vi "UHR-Fleezers Control (host) - Lorentz v4.vi"() -> ()   [LabVIEW 2014] (continued)
                                n2618 = Multiply(x=w4043, y=1000.0) -> (x*y=w4041:dbl)
                                n2619 = Wait (ms)(milliseconds to wait=w4041) -> ()  [unwired: 1 out]
                                }
                                frame #1 {
                                n2620 = local read "Yank to which?"() -> (w4045:bool)
                                n2621 = local read "Random Choice"() -> (w4055:bool)
                                n2622 = local read "Yank to Trap Delta (MHz)"() -> (w4048:dbl[])
                                n2623 = local read "Yank to SP"() -> (w4049:dbl[])
                                n2624 = Random Number (0-1)() -> (number: 0 to 1=w4054:dbl)
                                n2625 = Multiply(x=w4051, y=w4054) -> (x*y=w4053:dbl)
                                n2626 = Round Toward -Infinity(1:w4053) -> (0:w4052:dbl)
                                n2627 = Select(t=w4052, s=w4055, f=w4050) -> (s? t:f=w4046:dbl)
                                n2628 = Select(t=w4048, s=w4045, f=w4049) -> (s? t:f=w4047:dbl[])
                                n2629 = Index Array(array=w4047, index=w4046) -> (element=w4044:dbl)
                                n2630 = case shown="True" w4045 {
                                tunnel: w4044 -> [w4056 w4083]
                                frame False {
                                n2631 = flat-sequence {
                                tunnel: w4056 -> [w4057]
                                frame #0 {
                                n2632 = property on="Trap Pos FB SP" class="DigNum (strict)"("Val(Sgnl)"=w4057) -> ()  [unwired: 2 in, 2 out]
                                }
                                frame #1 {
                                n2633 = Wait (ms)(milliseconds to wait=u32 700) -> ()  [unwired: 1 out]
                                }
                                frame #2 {
                                n2634 = local read "Action (%)"() -> (w4062:dbl)
                                n2635 = Absolute Value(x=w4062) -> (abs(x)=w4061:dbl)
                                n2636 = Greater?(x=w4061, y=70.0) -> (0:w4059:bool)
                                n2637 = property on="Remove Action Offset" class="Bool (strict)"("Val(Sgnl)"=w4059) -> ()  [unwired: 2 in, 2 out]
                                }
                                frame #3 {
                                n2638 = for {
                                N: 4 -> [_]
                                n2639 = flat-sequence {
                                frame #0 {
                                n2640 = Wait (ms)(milliseconds to wait=u32 500) -> ()  [unwired: 1 out]
                                }
                                frame #1 {
                                n2641 = local read "Action (%)"() -> (w4068:dbl)
                                n2642 = Absolute Value(x=w4068) -> (abs(x)=w4067:dbl)
                                n2643 = Greater?(x=w4067, y=70.0) -> (0:w4065:bool)
                                n2644 = property on="Remove Action Offset" class="Bool (strict)"("Val(Sgnl)"=w4065) -> ()  [unwired: 2 in, 2 out]
                                }
                                }
                                }
                                }
                                frame #4 {
                                n2645 = Wait (ms)(milliseconds to wait=u32 500) -> ()  [unwired: 1 out]
                                }
                                frame #5 {
                                n2646 = local read "Mean"() -> (w4076:dbl)
                                n2647 = Greater?(x=w4076, y=11.0) -> (0:w4070:bool)
                                n2648 = Not(x=w4070) -> (.not. x?=w4071:bool)
                                n2649 = And(x=w4071, y="Shift confocal") -> (x .and. y?=w4073:bool)
                                n2650 = And(x=w4070, y="Shift confocal") -> (x .and. y?=w4074:bool)
                                n2651 = case shown="True" w4074 {
                                frame False {
                                }
                                frame True {
                                n2652 = local read "Confocal Y 2 (V)"() -> (w4080:dbl)
                                n2653 = local read "Confocal X 2 (V)"() -> (w4079:dbl)
                                n2654 = property on="AO1" class="Slide (strict)"("Val(Sgnl)"=w4080) -> ()  [unwired: 2 in, 2 out]
                                n2655 = property on="AO2" class="Slide (strict)"("Val(Sgnl)"=w4079) -> ()  [unwired: 2 in, 2 out]
                                }
                                }
                                n2656 = case shown="True" w4073 {
                                frame False {
                                }
                                frame True {
                                n2657 = local read "Confocal Y 1 (V)"() -> (w4078:dbl)
                                n2658 = local read "Confocal X 1 (V)"() -> (w4077:dbl)
                                n2659 = property on="AO1" class="Slide (strict)"("Val(Sgnl)"=w4078) -> ()  [unwired: 2 in, 2 out]
                                n2660 = property on="AO2" class="Slide (strict)"("Val(Sgnl)"=w4077) -> ()  [unwired: 2 in, 2 out]
                                }
                                }
                                }
                                frame #6 {
                                n2661 = Wait (ms)(milliseconds to wait=u32 1500) -> ()  [unwired: 1 out]
                                }
                                frame #7 {
                                n2662 = property on="Rem fb disp offset" class="Bool (strict)"("Val(Sgnl)"=TRUE ("Value (Signaling)")) -> ()  [unwired: 2 in, 2 out]
                                }
                                }
                                }
                                frame True {
                                n2663 = flat-sequence {
                                tunnel: w4083 -> [w4084]
                                frame #0 {
                                n2664 = property on="Trap Delta (MHz)" class="DigNum (strict)"("Val(Sgnl)"=w4084) -> ()  [unwired: 2 in, 2 out]
                                }
                                frame #1 {
                                n2665 = Wait (ms)(milliseconds to wait=u32 500) -> ()  [unwired: 1 out]
                                }
                                frame #2 {
                                n2666 = local read "Shift confocal"() -> (w4090:bool)
                                n2667 = local read "Mean"() -> (w4092:dbl)
                                n2668 = Greater?(x=w4092, y=11.0) -> (0:w4089:bool)
                                n2669 = Not(x=w4089) -> (.not. x?=w4088:bool)
                                n2670 = And(x=w4088, y=w4090) -> (x .and. y?=w4086:bool)
                                n2671 = And(x=w4089, y=w4090) -> (x .and. y?=w4087:bool)
                                n2672 = case shown="True" w4087 {
                                frame False {
                                }
                                frame True {
                                n2673 = local read "Confocal Y 2 (V)"() -> (w4096:dbl)
                                n2674 = local read "Confocal X 2 (V)"() -> (w4095:dbl)
                                n2675 = property on="AO2" class="Slide (strict)"("Val(Sgnl)"=w4095) -> ()  [unwired: 2 in, 2 out]
                                n2676 = property on="AO1" class="Slide (strict)"("Val(Sgnl)"=w4096) -> ()  [unwired: 2 in, 2 out]
                                }
                                }
                                n2677 = case shown="True" w4086 {
                                frame False {
                                }
                                frame True {
                                n2678 = local read "Confocal X 1 (V)"() -> (w4093:dbl)
                                n2679 = local read "Confocal Y 1 (V)"() -> (w4094:dbl)
                                n2680 = property on="AO2" class="Slide (strict)"("Val(Sgnl)"=w4093) -> ()  [unwired: 2 in, 2 out]
                                n2681 = property on="AO1" class="Slide (strict)"("Val(Sgnl)"=w4094) -> ()  [unwired: 2 in, 2 out]
                                }
                                }
                                }
                                }
                                }
                                }
                                }
                                }
                                }
                                frame "Image" {
                                n2682 = property on="Confocal Image" class="Bool (strict)"("Val(Sgnl)"=TRUE ("Value (Signaling)")) -> ()  [unwired: 2 in, 2 out]
                                }
                              }
                              n2683 = local write "Fl. High"(FALSE ("Fl. High")) -> ()
                              n2684 = local read "Time (s)"() -> (w4030:dbl)
                            }
                            frame #1 {
                              n2685 = case shown="True" "Auto F Reset" {
                                tunnel: w4102 -> [_ w4107]
                                tunnel: w4101 -> [_ w4106]
                                tunnel: w4100 -> [_ w4105]
                                tunnel: w4099 -> [_ w4104]
                                frame False {
                                }
                                frame True {
                                n2686 = node-c288() -> (w4109:T35)  [unwired: 4 in]
                                n2687 = timed-loop {
                                timing: w4109 -> [_]
                                timing-out: [_] -> w4108
                                tunnel: w4107 -> [w4114]
                                tunnel: w4106 -> [w4113]
                                tunnel: w4105 -> [w4112]
                                tunnel: w4104 -> [w4111]
                                stop <- w4110 stop-if-true
                                n2688 = node-c288() -> ()  [unwired: 1 in, 1 out]
                                n2689 = local read "Fl. Delta Thresh. (kHz)"() -> (w4123:dbl)
                                n2690 = local read "APD to Watch"() -> (w4124:bool)
                                n2691 = local read "Delta Fl. 1"() -> (w4125:dbl)
                                n2692 = local read "Delta Fl. 2"() -> (w4126:dbl)
                                n2693 = local read "Fl. Triggered..."() -> (w4117:bool)
                                n2694 = local read "Stop All"() -> (w4118:bool)
                                n2695 = local read "Reset Force"() -> (w4116:bool)
                                n2696 = Multiply(x=w4123, y=1000.0) -> (x*y=w4121:dbl)
                                n2697 = Select(t=w4125, s=w4124, f=w4126) -> (s? t:f=w4120:dbl)
                                n2698 = Not(x=w4117) -> (.not. x?=w4115:bool)
                                n2699 = Greater?(x=w4120, y=w4121) -> (0:w4119:bool)
                                n2700 = Compound Arithmetic op=OR(w4119, w4118, w4115, w4116) -> (w4110:bool)
                                n2701 = case shown="True" w4110 {
                                tunnel: w4114 -> [_ w4130]
                                tunnel: w4113 -> [_ w4134]
                                tunnel: w4112 -> [_ w4133]
                                tunnel: w4111 -> [_ w4132]
                                frame False {
                                }
                                frame True {
                                n2702 = case shown="\"Yank\"" w4134 {
                                tunnel: w4133 -> [_ w4144]
                                tunnel: w4132 -> [_ w4142]
                                frame "Image", Default {
                                }
                                frame "Yank" {
                                n2703 = flat-sequence {
                                tunnel: [w4147] -> w4145
                                tunnel: w4144 -> [w4147]
                                tunnel: [w4146] -> w4143
                                tunnel: w4142 -> [w4146]
                                tunnel: w4145 -> [w4153]
                                tunnel: w4143 -> [w4151]
                                frame #0 {
                                n2704 = local read "Yank Delay (s)"() -> (w4150:dbl)
                                n2705 = Multiply(x=w4150, y=1000.0) -> (x*y=w4148:dbl)
                                n2706 = Wait (ms)(milliseconds to wait=w4148) -> ()  [unwired: 1 out]
                                }
                                frame #1 {
                                n2707 = local read "Yank to which?"() -> (w4152:bool)
                                n2708 = case shown="False" w4152 {
                                tunnel: w4153 -> [_ w4181]
                                tunnel: w4151 -> [w4154 _]
                                frame False {
                                n2709 = flat-sequence {
                                tunnel: w4154 -> [w4155]
                                frame #0 {
                                n2710 = property on="Trap Pos FB SP" class="DigNum (strict)"("Val(Sgnl)"=w4155) -> ()  [unwired: 2 in, 2 out]
                                }
                                frame #1 {
                                n2711 = Wait (ms)(milliseconds to wait=u32 700) -> ()  [unwired: 1 out]
                                }
                                frame #2 {
                                n2712 = local read "Action (%)"() -> (w4160:dbl)
                                n2713 = Absolute Value(x=w4160) -> (abs(x)=w4159:dbl)
                                n2714 = Greater?(x=w4159, y=70.0) -> (0:w4157:bool)
                                n2715 = property on="Remove Action Offset" class="Bool (strict)"("Val(Sgnl)"=w4157) -> ()  [unwired: 2 in, 2 out]
                                }
                                frame #3 {
                                n2716 = for {
                                N: 4 -> [_]
                                n2717 = flat-sequence {
                                frame #0 {
                                n2718 = Wait (ms)(milliseconds to wait=u32 500) -> ()  [unwired: 1 out]
                                }
                                frame #1 {
                                n2719 = local read "Action (%)"() -> (w4166:dbl)
                                n2720 = Absolute Value(x=w4166) -> (abs(x)=w4165:dbl)
                                n2721 = Greater?(x=w4165, y=70.0) -> (0:w4163:bool)
                                n2722 = property on="Remove Action Offset" class="Bool (strict)"("Val(Sgnl)"=w4163) -> ()  [unwired: 2 in, 2 out]
                                }
                                }
                                }
                                }
                                frame #4 {
                                n2723 = Wait (ms)(milliseconds to wait=u32 500) -> ()  [unwired: 1 out]
                                }
                                frame #5 {
                                n2724 = local read "Shift confocal"() -> (w4171:bool)
                                n2725 = local read "Mean"() -> (w4174:dbl)
                                n2726 = Greater?(x=w4174, y=11.0) -> (0:w4170:bool)
                                n2727 = Not(x=w4170) -> (.not. x?=w4169:bool)
                                n2728 = And(x=w4170, y=w4171) -> (x .and. y?=w4172:bool)
                                n2729 = And(x=w4169, y=w4171) -> (x .and. y?=w4168:bool)
                                n2730 = case shown="True" w4172 {
                                frame False {
                                }
                                frame True {
                                n2731 = local read "Confocal X 2 (V)"() -> (w4177:dbl)
                                n2732 = local read "Confocal Y 2 (V)"() -> (w4178:dbl)
                                n2733 = property on="AO2" class="Slide (strict)"("Val(Sgnl)"=w4177) -> ()  [unwired: 2 in, 2 out]
                                n2734 = property on="AO1" class="Slide (strict)"("Val(Sgnl)"=w4178) -> ()  [unwired: 2 in, 2 out]
                                }
                                }
                                n2735 = case shown="True" w4168 {
                                frame False {
                                }
                                frame True {
                                n2736 = local read "Confocal Y 1 (V)"() -> (w4176:dbl)
                                n2737 = local read "Confocal X 1 (V)"() -> (w4175:dbl)
                                n2738 = property on="AO1" class="Slide (strict)"("Val(Sgnl)"=w4176) -> ()  [unwired: 2 in, 2 out]
                                n2739 = property on="AO2" class="Slide (strict)"("Val(Sgnl)"=w4175) -> ()  [unwired: 2 in, 2 out]
                                }
                                }
                                }
                                frame #6 {
                                n2740 = Wait (ms)(milliseconds to wait=u32 1500) -> ()  [unwired: 1 out]
                                }
                                frame #7 {
                                n2741 = property on="Rem fb disp offset" class="Bool (strict)"("Val(Sgnl)"=TRUE ("Value (Signaling)")) -> ()  [unwired: 2 in, 2 out]
                                }
                                }
                                }
                                frame True {
                                n2742 = flat-sequence {
                                tunnel: w4181 -> [w4182]
                                frame #0 {
                                n2743 = property on="Trap Delta (MHz)" class="DigNum (strict)"("Val(Sgnl)"=w4182) -> ()  [unwired: 2 in, 2 out]
                                }
                                frame #1 {
                                n2744 = Wait (ms)(milliseconds to wait=u32 500) -> ()  [unwired: 1 out]
                                }
                                frame #2 {
                                n2745 = local read "Shift confocal"() -> (w4188:bool)
                                n2746 = local read "Mean"() -> (w4189:dbl)
                                n2747 = Greater?(x=w4189, y=11.0) -> (0:w4187:bool)
                                n2748 = And(x=w4187, y=w4188) -> (x .and. y?=w4185:bool)
                                n2749 = Not(x=w4187) -> (.not. x?=w4186:bool)
                                n2750 = And(x=w4186, y=w4188) -> (x .and. y?=w4184:bool)
                                n2751 = case shown="True" w4185 {
                                frame False {
                                }
                                frame True {
                                n2752 = local read "Confocal Y 2 (V)"() -> (w4194:dbl)
                                n2753 = local read "Confocal X 2 (V)"() -> (w4193:dbl)
                                n2754 = property on="AO1" class="Slide (strict)"("Val(Sgnl)"=w4194) -> ()  [unwired: 2 in, 2 out]
                                n2755 = property on="AO2" class="Slide (strict)"("Val(Sgnl)"=w4193) -> ()  [unwired: 2 in, 2 out]
                                }
                                }
                                n2756 = case shown="True" w4184 {
                                frame False {
                                }
                                frame True {
                                n2757 = local read "Confocal Y 1 (V)"() -> (w4192:dbl)
                                n2758 = local read "Confocal X 1 (V)"() -> (w4191:dbl)
                                n2759 = property on="AO2" class="Slide (strict)"("Val(Sgnl)"=w4191) -> ()  [unwired: 2 in, 2 out]
                                n2760 = property on="AO1" class="Slide (strict)"("Val(Sgnl)"=w4192) -> ()  [unwired: 2 in, 2 out]
                                }
                                }
                                }
                                }
                                }
                                }
                                }
                                }
                                }
                                }
                                n2761 = local read "Time (s)"() -> (w4129:dbl)
                                n2762 = Subtract(x=w4130, y=w4129) -> (x-y=w4141:dbl)
                                n2763 = Number To Decimal String(number=w4141, width (-)=i16 0) -> (decimal integer string=w4139:string)
                                n2764 = Concatenate Strings(w4139, " s fluorescence event") -> (w4136:string)
                                n2765 = local read "Messages"() -> (w4137:string)
                                n2766 = local write "Duration (s)"(w4141) -> ()
                                n2767 = call "Update messages.vi"("Message to add"=w4136, "Old message string"=w4137) -> ("New message string"=w4135:string)
                                n2768 = local write "Messages"(w4135) -> ()
                                n2769 = call <vilib>:"Beep.vi"() -> ()  [unwired: 12 in]
                                n2770 = local write "Reset Force"(FALSE ("Force Reset")) -> ()
                                n2771 = local write "Fl. High"(TRUE ("Fl. High")) -> ()
                                n2772 = local write "Waiting"(TRUE ("Waiting")) -> ()
                                }
                                }
                                n2773 = node-c288() -> ()  [unwired: 1 in, 1 out]
                                }
                                n2774 = node-c288(w4108) -> ()  [unwired: 1 out]
                                }
                              }
                            }
                          }
                          n2775 = local read "Trap Delta (MHz)"() -> (w4020:dbl)
                          n2776 = local read "Trap Pos FB SP"() -> (w4018:fxp<+/-,16,1>)
                        }
                      }
                    }
                    frame True {
                      n2777 = flat-sequence {
                        tunnel: w4205 -> [w4215]
                        tunnel: [w4215] -> w4209
                        tunnel: w4208 -> [w4214]
                        tunnel: [w4214] -> w4207
                        tunnel: [w4213] -> w4206
                        tunnel: w4204 -> [w4212]
                        tunnel: [w4211] -> w4203
                        tunnel: w4200 -> [w4210]
                        tunnel: [w4210] -> w4199
                        tunnel: w4209 -> [w4285]
                        tunnel: w4207 -> [w4284]
                        tunnel: w4206 -> [w4283]
                        tunnel: w4203 -> [w4282]
                        tunnel: w4199 -> [w4281]
                        tunnel: [w4282] -> w4202
                        frame #0 {
                          n2778 = call <vilib>:"Beep.vi"() -> ()  [unwired: 3 in, 9 out]
                          n2779 = local write "Waiting"(FALSE ("Waiting")) -> ()
                          n2780 = Increment(x=w4212) -> (x+1=w4211:u8)
                          n2781 = case shown="\"Image\"" w4214 {
                            tunnel: w4211 -> [_ _ w4221]
                            frame "Image" {
                              n2782 = property on="Confocal Image" class="Bool (strict)"("Val(Sgnl)"=TRUE ("Value (Signaling)")) -> ()  [unwired: 2 in, 2 out]
                            }
                            frame "Alarm", Default {
                            }
                            frame "Yank" {
                              n2783 = flat-sequence {
                                tunnel: w4221 -> [w4224]
                                tunnel: [w4223] -> w4220
                                tunnel: ["N Array El"] -> w4219
                                tunnel: w4220 -> [w4238]
                                tunnel: w4219 -> [w4234]
                                frame #0 {
                                n2784 = Multiply(x="Yank Delay (s)", y=1000.0) -> (x*y=w4227:dbl)
                                n2785 = Quotient & Remainder(x=w4224, y="N Array El") -> (x-y*floor(x/y)=w4223:u8)  [unwired: 1 out]
                                n2786 = Wait (ms)(milliseconds to wait=w4227) -> ()  [unwired: 1 out]
                                }
                                frame #1 {
                                n2787 = Random Number (0-1)() -> (number: 0 to 1=w4235:dbl)
                                n2788 = Multiply(x=w4234, y=w4235) -> (x*y=w4233:dbl)
                                n2789 = Round Toward -Infinity(1:w4233) -> (0:w4232:dbl)
                                n2790 = Select(t=w4232, s="Random Choice", f=w4238) -> (s? t:f=w4236:dbl)
                                n2791 = Select(t="Yank to Trap Delta (MHz)", s="Yank to which?", f="Yank to SP") -> (s? t:f=w4229:dbl[])
                                n2792 = Index Array(array=w4229, index=w4236) -> (element=w4239:dbl)
                                n2793 = case shown="False" "Yank to which?" {
                                tunnel: w4239 -> [w4240 w4266]
                                frame False {
                                n2794 = flat-sequence {
                                tunnel: w4240 -> [w4241]
                                frame #0 {
                                n2795 = property on="Trap Pos FB SP" class="DigNum (strict)"("Val(Sgnl)"=w4241) -> ()  [unwired: 2 in, 2 out]
                                }
                                frame #1 {
                                n2796 = Wait (ms)(milliseconds to wait=u32 700) -> ()  [unwired: 1 out]
                                }
                                frame #2 {
                                n2797 = local read "Action (%)"() -> (w4246:dbl)
                                n2798 = Absolute Value(x=w4246) -> (abs(x)=w4245:dbl)
                                n2799 = Greater?(x=w4245, y=70.0) -> (0:w4243:bool)
                                n2800 = property on="Remove Action Offset" class="Bool (strict)"("Val(Sgnl)"=w4243) -> ()  [unwired: 2 in, 2 out]
                                }
                                frame #3 {
                                n2801 = for {
                                N: 4 -> [_]
                                n2802 = flat-sequence {
                                frame #0 {
                                n2803 = Wait (ms)(milliseconds to wait=u32 500) -> ()  [unwired: 1 out]
                                }
                                frame #1 {
                                n2804 = local read "Action (%)"() -> (w4252:dbl)
                                n2805 = Absolute Value(x=w4252) -> (abs(x)=w4251:dbl)
                                n2806 = Greater?(x=w4251, y=70.0) -> (0:w4249:bool)
                                n2807 = property on="Remove Action Offset" class="Bool (strict)"("Val(Sgnl)"=w4249) -> ()  [unwired: 2 in, 2 out]
                                }
                                }
                                }
                                }
                                frame #4 {
                                n2808 = local read "Shift confocal"() -> (w4256:bool)
                                n2809 = local read "Mean"() -> (w4259:dbl)
                                n2810 = Greater?(x=w4259, y=11.0) -> (0:w4255:bool)
                                n2811 = Not(x=w4255) -> (.not. x?=w4254:bool)
                                n2812 = And(x=w4254, y=w4256) -> (x .and. y?=w4253:bool)
                                n2813 = And(x=w4255, y=w4256) -> (x .and. y?=w4257:bool)
                                n2814 = case shown="True" w4257 {
                                frame False {
                                }
                                frame True {
                                n2815 = local read "Confocal X 2 (V)"() -> (w4262:dbl)
                                n2816 = local read "Confocal Y 2 (V)"() -> (w4263:dbl)
                                n2817 = property on="AO2" class="Slide (strict)"("Val(Sgnl)"=w4262) -> ()  [unwired: 2 in, 2 out]
                                n2818 = property on="AO1" class="Slide (strict)"("Val(Sgnl)"=w4263) -> ()  [unwired: 2 in, 2 out]
                                }
                                }
                                n2819 = case shown="True" w4253 {
                                frame False {
                                }
                                frame True {
                                n2820 = local read "Confocal X 1 (V)"() -> (w4260:dbl)
                                n2821 = local read "Confocal Y 1 (V)"() -> (w4261:dbl)
                                n2822 = property on="AO1" class="Slide (strict)"("Val(Sgnl)"=w4261) -> ()  [unwired: 2 in, 2 out]
                                n2823 = property on="AO2" class="Slide (strict)"("Val(Sgnl)"=w4260) -> ()  [unwired: 2 in, 2 out]
                                }
                                }
                                }
                                frame #5 {
                                n2824 = Wait (ms)(milliseconds to wait=u32 1500) -> ()  [unwired: 1 out]
                                }
                                frame #6 {
                                n2825 = property on="Rem fb disp offset" class="Bool (strict)"("Val(Sgnl)"=TRUE ("Value (Signaling)")) -> ()  [unwired: 2 in, 2 out]
                                }
                                }
                                }
                                frame True {
                                n2826 = flat-sequence {
                                tunnel: w4266 -> [w4267]
                                frame #0 {
                                n2827 = property on="Trap Delta (MHz)" class="DigNum (strict)"("Val(Sgnl)"=w4267) -> ()  [unwired: 2 in, 2 out]
                                }
                                frame #1 {
                                n2828 = Wait (ms)(milliseconds to wait=u32 500) -> ()  [unwired: 1 out]
                                }
                                frame #2 {
                                n2829 = local read "Shift confocal"() -> (w4271:bool)
                                n2830 = local read "Mean"() -> (w4269:dbl)
                                n2831 = Greater?(x=w4269, y=11.0) -> (0:w4272:bool)
                                n2832 = Not(x=w4272) -> (.not. x?=w4273:bool)
                                n2833 = And(x=w4273, y=w4271) -> (x .and. y?=w4275:bool)
                                n2834 = And(x=w4272, y=w4271) -> (x .and. y?=w4274:bool)
                                n2835 = case shown="True" w4274 {
                                frame False {
                                }
                                frame True {
                                n2836 = local read "Confocal Y 2 (V)"() -> (w4279:dbl)
                                n2837 = local read "Confocal X 2 (V)"() -> (w4278:dbl)
                                n2838 = property on="AO1" class="Slide (strict)"("Val(Sgnl)"=w4279) -> ()  [unwired: 2 in, 2 out]
                                n2839 = property on="AO2" class="Slide (strict)"("Val(Sgnl)"=w4278) -> ()  [unwired: 2 in, 2 out]
                                }
                                }
                                n2840 = case shown="True" w4275 {
                                frame False {
                                }
                                frame True {
                                n2841 = local read "Confocal X 1 (V)"() -> (w4276:dbl)
                                n2842 = local read "Confocal Y 1 (V)"() -> (w4277:dbl)
                                n2843 = property on="AO2" class="Slide (strict)"("Val(Sgnl)"=w4276) -> ()  [unwired: 2 in, 2 out]
                                n2844 = property on="AO1" class="Slide (strict)"("Val(Sgnl)"=w4277) -> ()  [unwired: 2 in, 2 out]
                                }
                                }
                                }
                                }
                                }
                                }
                                }
                              }
                            }
                          }
                          n2845 = local read "Time (s)"() -> (w4213:dbl)
                          "Fl. High" <- TRUE ("Yanking")
                        }
                        frame #1 {
                          n2846 = local read "Auto F Reset"() -> (w4280:bool)
                          n2847 = case shown="True" w4280 {
                            tunnel: w4285 -> [_ w4289]
                            tunnel: w4284 -> [_ w4288]
                            tunnel: w4283 -> [_ w4287]
                            tunnel: w4281 -> [_ w4286]
                            frame False {
                            }
                            frame True {
                              n2848 = node-c288() -> (w4291:T35)  [unwired: 4 out]
                              n2849 = timed-loop {
                                timing: w4291 -> [_]
                                timing-out: [_] -> w4290
                                tunnel: w4289 -> [w4309]
                                tunnel: w4288 -> [w4308]
                                tunnel: w4287 -> [w4307]
                                tunnel: w4286 -> [w4306]
                                stop <- w4292 stop-if-true
                                n2850 = node-c288() -> ()  [unwired: 2 out]
                                n2851 = local read "Fl. Delta Thresh. (kHz)"() -> (w4300:dbl)
                                n2852 = local read "Fl. Triggered..."() -> (w4305:bool)
                                n2853 = local read "Delta Fl. 1"() -> (w4296:dbl)
                                n2854 = local read "Delta Fl. 2"() -> (w4294:dbl)
                                n2855 = local read "Stop All"() -> (w4303:bool)
                                n2856 = local read "APD to Watch"() -> (w4295:bool)
                                n2857 = Select(t=w4296, s=w4295, f=w4294) -> (s? t:f=w4293:dbl)
                                n2858 = Not(x=w4305) -> (.not. x?=w4304:bool)
                                n2859 = Multiply(x=w4300, y=1000.0) -> (x*y=w4299:dbl)
                                n2860 = Negate(x=w4299) -> (-x=w4298:dbl)
                                n2861 = Less?(x=w4293, y=w4298) -> (x < y?=w4302:bool)
                                n2862 = Compound Arithmetic op=OR(w4302, w4303, w4304, "Reset Force") -> (w4292:bool)
                                n2863 = case shown="True" w4292 {
                                tunnel: w4309 -> [_ w4324]
                                tunnel: w4308 -> [_ w4323]
                                tunnel: w4307 -> [_ w4313]
                                tunnel: w4306 -> [_ w4315]
                                frame False {
                                }
                                frame True {
                                n2864 = local read "Time (s)"() -> (w4314:dbl)
                                n2865 = case shown="\"Yank\"" w4323 {
                                tunnel: w4324 -> [_ w4327]
                                tunnel: w4315 -> [_ w4325]
                                frame "Image", Default {
                                }
                                frame "Yank" {
                                n2866 = flat-sequence {
                                tunnel: [w4333] -> w4328
                                tunnel: w4327 -> [w4333]
                                tunnel: [w4329] -> w4326
                                tunnel: w4325 -> [w4329]
                                tunnel: w4328 -> [w4336]
                                tunnel: w4326 -> [w4334]
                                frame #0 {
                                n2867 = local read "Yank Delay (s)"() -> (w4332:dbl)
                                n2868 = Multiply(x=w4332, y=1000.0) -> (x*y=w4330:dbl)
                                n2869 = Wait (ms)(milliseconds to wait=w4330) -> ()  [unwired: 1 out]
                                }
                                frame #1 {
                                n2870 = local read "Yank to which?"() -> (w4335:bool)
                                n2871 = case shown="False" w4335 {
                                tunnel: w4336 -> [_ w4363]
                                tunnel: w4334 -> [w4337 _]
                                frame False {
                                n2872 = flat-sequence {
                                tunnel: w4337 -> [w4338]
                                frame #0 {
                                n2873 = property on="Trap Pos FB SP" class="DigNum (strict)"("Val(Sgnl)"=w4338) -> ()  [unwired: 2 in, 2 out]
                                }
                                frame #1 {
                                n2874 = Wait (ms)(milliseconds to wait=u32 700) -> ()  [unwired: 1 out]
                                }
                                frame #2 {
                                n2875 = local read "Action (%)"() -> (w4343:dbl)
                                n2876 = Absolute Value(x=w4343) -> (abs(x)=w4342:dbl)
                                n2877 = Greater?(x=w4342, y=70.0) -> (0:w4340:bool)
                                n2878 = property on="Remove Action Offset" class="Bool (strict)"("Val(Sgnl)"=w4340) -> ()  [unwired: 2 in, 2 out]
                                }
                                frame #3 {
                                n2879 = for {
                                N: 4 -> [_]
                                n2880 = flat-sequence {
                                frame #0 {
                                n2881 = Wait (ms)(milliseconds to wait=u32 500) -> ()  [unwired: 1 out]
                                }
                                frame #1 {
                                n2882 = local read "Action (%)"() -> (w4349:dbl)
                                n2883 = Absolute Value(x=w4349) -> (abs(x)=w4348:dbl)
                                n2884 = Greater?(x=w4348, y=70.0) -> (0:w4346:bool)
                                n2885 = property on="Remove Action Offset" class="Bool (strict)"("Val(Sgnl)"=w4346) -> ()  [unwired: 2 in, 2 out]
                                }
                                }
                                }
                                }
                                frame #4 {
                                n2886 = local read "Shift confocal"() -> (w4354:bool)
                                n2887 = local read "Mean"() -> (w4356:dbl)
                                n2888 = Greater?(x=w4356, y=11.0) -> (0:w4353:bool)
                                n2889 = Not(x=w4353) -> (.not. x?=w4352:bool)
                                n2890 = And(x=w4353, y=w4354) -> (x .and. y?=w4351:bool)
                                n2891 = And(x=w4352, y=w4354) -> (x .and. y?=w4350:bool)
                                n2892 = case shown="True" w4351 {
                                frame False {
                                }
                                frame True {
                                n2893 = local read "Confocal Y 2 (V)"() -> (w4360:dbl)
                                n2894 = local read "Confocal X 2 (V)"() -> (w4359:dbl)
                                n2895 = property on="AO2" class="Slide (strict)"("Val(Sgnl)"=w4359) -> ()  [unwired: 2 in, 2 out]
                                n2896 = property on="AO1" class="Slide (strict)"("Val(Sgnl)"=w4360) -> ()  [unwired: 2 in, 2 out]
                                }
                                }
                                n2897 = case shown="True" w4350 {
                                frame False {
                                }
                                frame True {
                                n2898 = local read "Confocal X 1 (V)"() -> (w4357:dbl)
                                n2899 = local read "Confocal Y 1 (V)"() -> (w4358:dbl)
                                n2900 = property on="AO1" class="Slide (strict)"("Val(Sgnl)"=w4358) -> ()  [unwired: 2 in, 2 out]
                                n2901 = property on="AO2" class="Slide (strict)"("Val(Sgnl)"=w4357) -> ()  [unwired: 2 in, 2 out]
                                }
                                }
                                }
                                frame #5 {
                                n2902 = Wait (ms)(milliseconds to wait=u32 1500) -> ()  [unwired: 1 out]
                                }
                                frame #6 {
                                n2903 = property on="Rem fb disp offset" class="Bool (strict)"("Val(Sgnl)"=TRUE ("Value (Signaling)")) -> ()  [unwired: 2 in, 2 out]
                                }
                                }
                                }
                                frame True {
                                n2904 = flat-sequence {
                                tunnel: w4363 -> [w4364]
                                frame #0 {
                                n2905 = property on="Trap Delta (MHz)" class="DigNum (strict)"("Val(Sgnl)"=w4364) -> ()  [unwired: 2 in, 2 out]
                                }
                                frame #1 {
                                n2906 = Wait (ms)(milliseconds to wait=u32 500) -> ()  [unwired: 1 out]
                                }
                                frame #2 {
                                n2907 = local read "Shift confocal"() -> (w4370:bool)
                                n2908 = local read "Mean"() -> (w4372:dbl)
                                n2909 = Greater?(x=w4372, y=11.0) -> (0:w4369:bool)
                                n2910 = Not(x=w4369) -> (.not. x?=w4368:bool)
                                n2911 = And(x=w4369, y=w4370) -> (x .and. y?=w4367:bool)
                                n2912 = And(x=w4368, y=w4370) -> (x .and. y?=w4366:bool)
                                n2913 = case shown="True" w4367 {
                                frame False {
                                }
                                frame True {
                                n2914 = local read "Confocal Y 2 (V)"() -> (w4376:dbl)
                                n2915 = local read "Confocal X 2 (V)"() -> (w4375:dbl)
                                n2916 = property on="AO2" class="Slide (strict)"("Val(Sgnl)"=w4375) -> ()  [unwired: 2 in, 2 out]
                                n2917 = property on="AO1" class="Slide (strict)"("Val(Sgnl)"=w4376) -> ()  [unwired: 2 in, 2 out]
                                }
                                }
                                n2918 = case shown="True" w4366 {
                                frame False {
                                }
                                frame True {
                                n2919 = local read "Confocal Y 1 (V)"() -> (w4374:dbl)
                                n2920 = local read "Confocal X 1 (V)"() -> (w4373:dbl)
                                n2921 = property on="AO2" class="Slide (strict)"("Val(Sgnl)"=w4373) -> ()  [unwired: 2 in, 2 out]
                                n2922 = property on="AO1" class="Slide (strict)"("Val(Sgnl)"=w4374) -> ()  [unwired: 2 in, 2 out]
                                }
                                }
                                }
                                }
                                }
                                }
                                }
                                }
                                }
                                }
                                n2923 = local read "Messages"() -> (w4322:string)
                                n2924 = Subtract(x=w4314, y=w4313) -> (x-y=w4320:dbl)
                                "Duration (s)" <- w4320
                                n2925 = Number To Decimal String(number=w4320, width (-)=i16 0) -> (decimal integer string=w4318:string)
                                n2926 = Concatenate Strings(w4318, " s fluorescence event." ("string")) -> (w4316:string)
                                n2927 = call "Update messages.vi"("Message to add"=w4316, "Old message string"=w4322) -> ("New message string"=w4321:string)
                                n2928 = local write "Reset Force"(FALSE ("Reset Force")) -> ()
                                n2929 = local write "Waiting"(TRUE ("Waiting")) -> ()
                                n2930 = local write "Messages"(w4321) -> ()
                                n2931 = local write "Fl. High"(FALSE ("Fl. High")) -> ()
                                n2932 = call <vilib>:"Beep.vi"() -> ()  [unwired: 3 in, 9 out]
                                }
                                }
                                n2933 = node-c288() -> ()  [unwired: 2 out]
                              }
                              n2934 = node-c288(w4290) -> ()  [unwired: 1 out]
                            }
                          }
                        }
                      }
                      n2935 = local read "Trap Delta (MHz)"() -> (w4205:dbl)
                      n2936 = local read "Trap Pos FB SP"() -> (w4200:fxp<+/-,16,1>)
                    }
                  }
                }
                frame #1 {
                  n2937 = local read "Stop All"() -> (w4386:bool)
                  n2938 = local read "Fl. Triggered..."() -> (w4384:bool)
                  n2939 = Not(x=w4384) -> (.not. x?=w4385:bool)
                  n2940 = Or(x=w4385, y=w4386) -> (x .or. y?=w4383:bool)
                }
              }
              n2941 = case shown="True" w3977 {
                frame False {
                }
                frame True {
                  n2942 = local read "Confocal Y 1 (V)"() -> (w3987:dbl)
                  n2943 = local read "Confocal X 1 (V)"() -> (w3986:dbl)
                  n2944 = property on="AO2" class="Slide (strict)"("Val(Sgnl)"=w3986) -> ()  [unwired: 2 in, 2 out]
                  n2945 = property on="AO1" class="Slide (strict)"("Val(Sgnl)"=w3987) -> ()  [unwired: 2 in, 2 out]
                }
              }
              n2946 = case shown="True" w3977 {
                frame False {
                }
                frame True {
                  w3985 = FALSE ("Fl. High")
                  n2947 = local write "Waiting"(w3985) -> ()
                  n2948 = local write "Fl. High"(w3985) -> ()
                }
              }
              n2949 = node-c288() -> ()  [unwired: 2 out]
            }
            n2950 = node-c288(w3975) -> ()  [unwired: 1 out]
          }
        }
      }
      event "Start assembly line": Value Change {
        n2951 = event-data() -> ()  [unwired: 7 out]
        n2952 = case shown="True" "Start assembly line" {
          tunnel: w4392 -> [_ w4393]
          frame False {
          }
          frame True {
            n2953 = flat-sequence {
              tunnel: w4393 -> [w4398]
              tunnel: [w4397] -> w4395
              tunnel: w4395 -> [w4430]
              tunnel: [w4429] -> w4394
              tunnel: w4394 -> [w4432]
              tunnel: w4393 -> [w4451]
              frame #0 {
                w4396 = TRUE ("Value (Signaling)")
                n2954 = property on="Green Laser ON" class="Bool (strict)"("Val(Sgnl)"=w4396) -> ()  [unwired: 2 in, 2 out]
                "AL Running" <- w4396
              }
              frame #1 {
                n2955 = node-c288() -> (w4400:T35)  [unwired: 4 in]
                n2956 = timed-loop {
                  timing: w4400 -> [_]
                  timing-out: [_] -> w4399
                  tunnel: w4398 -> [w4408]
                  tunnel: [w4403] -> w4397
                  stop <- w4404 stop-if-true
                  n2957 = node-c288() -> ()  [unwired: 1 in, 1 out]
                  n2958 = local read "APD rates cluster"() -> (w4402:T2)
                  n2959 = Multiply(x="Cy3 Fl.  Thresh. (kHz)", y=1000.0) -> (x*y=w4411:dbl)
                  n2960 = Unbundle By Name(w4402) -> ("APD 1 Rate (Hz)"=w4401:dbl)
                  n2961 = Greater?(x=w4401, y=w4411) -> (0:w4407:bool)
                  n2962 = case shown="True" w4407 {
                    tunnel: w4408 -> [_ w4414]
                    tunnel: [TRUE ("Stage Moving") w4413] -> w4406
                    frame False {
                    }
                    frame True {
                      n2963 = flat-sequence {
                        tunnel: w4414 -> [w4419]
                        tunnel: [w4424] -> w4413
                        frame #0 {
                          n2964 = Multiply(x="AL Delay (s)", y=u32 1000) -> (x*y=w4416:u32)
                          n2965 = Wait (ms)(milliseconds to wait=w4416) -> ()  [unwired: 1 out]
                        }
                        frame #1 {
                          n2966 = property on="Green Laser ON" class="Bool (strict)"("Val(Sgnl)"=FALSE ("Value (Signaling)")) -> ()  [unwired: 2 in, 2 out]
                        }
                        frame #2 {
                          # "upper spot"
                          n2967 = local read "Saved Stage Positions"() -> (w4422:dbl[][])
                          n2968 = local write "Stage Moving"(TRUE ("Stage Moving")) -> ()
                          n2969 = call "move to saved stage position.vi"("Stage VISA resource name in"=w4419, "Position"=5, "Saved Stage Positions"=w4422) -> ("error out"=w4420:errorcluster)  [unwired: 1 in, 1 out]
                          n2970 = local write "Stage Control Serial Error"(w4420) -> ()
                        }
                        frame #3 {
                          w4424 = FALSE ("Stage Moving")
                          n2971 = call <vilib>:"Beep.vi"() -> ()  [unwired: 3 in, 9 out]
                          n2972 = local write "Stage Moving"(w4424) -> ()
                        }
                      }
                    }
                  }
                  n2973 = local read "Stop assembly line"() -> (w4403:bool)
                  n2974 = Not(x=w4406) -> (.not. x?=w4405:bool)
                  n2975 = node-c288() -> ()  [unwired: 1 in, 1 out]
                  n2976 = Or(x=w4405, y=w4403) -> (x .or. y?=w4404:bool)
                }
                n2977 = node-c288(w4399) -> ()  [unwired: 1 out]
              }
              frame #2 {
                n2978 = Not(x=w4430) -> (.not. x?=w4429:bool)
                n2979 = case shown="True" w4429 {
                  frame False {
                  }
                  frame True {
                    n2980 = property on="Red Laser ON" class="Bool (strict)"("Val(Sgnl)"=TRUE ("Value (Signaling)")) -> ()  [unwired: 2 in, 2 out]
                  }
                }
              }
              frame #3 {
                n2981 = node-c288() -> (w4434:T35)  [unwired: 4 in]
                n2982 = timed-loop {
                  timing: w4434 -> [_]
                  timing-out: [_] -> w4433
                  tunnel: [w4437] -> _
                  tunnel: w4432 -> [w4437]
                  stop <- "Stop assembly line" stop-if-true
                  n2983 = node-c288() -> ()  [unwired: 1 in, 1 out]
                  n2984 = local read "APD rates cluster"() -> (w4436:T2)
                  n2985 = Multiply(x="Cy5 Fl.  Thresh. (kHz)", y=1000.0) -> (x*y=w4443:dbl)
                  n2986 = Unbundle By Name(w4436) -> ("APD 2 Rate (Hz)"=w4435:dbl)
                  n2987 = Greater?(x=w4435, y=w4443) -> (0:w4440:bool)
                  n2988 = And(x=w4440, y=w4437) -> (x .and. y?=w4438:bool)
                  n2989 = case shown="True" w4438 {
                    frame False {
                    }
                    frame True {
                      n2990 = property on="Green Laser ON" class="Bool (strict)"("Val(Sgnl)"=TRUE ("Value (Signaling)")) -> ()  [unwired: 2 in, 2 out]
                    }
                  }
                  n2991 = node-c288() -> ()  [unwired: 1 in, 1 out]
                }
                n2992 = node-c288(w4433) -> ()  [unwired: 1 out]
              }
              frame #4 {
                w4450 = FALSE ("Value (Signaling)")
                # "lower spot"
                n2993 = local read "Saved Stage Positions"() -> (w4454:dbl[][])
                n2994 = property on="Red Laser ON" class="Bool (strict)"("Val(Sgnl)"=w4450) -> ()  [unwired: 2 in, 2 out]
                n2995 = property on="Green Laser ON" class="Bool (strict)"("Val(Sgnl)"=w4450) -> ()  [unwired: 2 in, 2 out]
                n2996 = local write "Stage Moving"(TRUE ("Stage Moving")) -> ()
                n2997 = local write "Stop assembly line"(FALSE ("Stop assembly line")) -> ()
